vi "LWXPS_Example_GatheringCurrentNumberGet.vi"() -> ()   [LabVIEW 2013]
panel:
  out "Error out":errorcluster caption="error out"
  out "Current Number":i32
  out "Maximum Samples Number":i32
  in  "Instrument Key IN":string
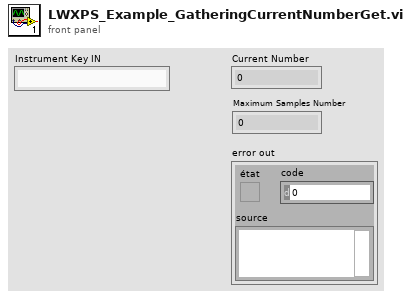
[diagram p1: front panel]
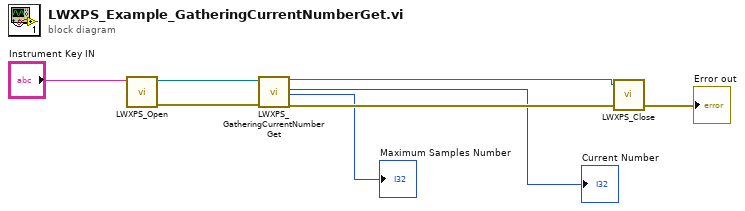
[diagram p0: block diagram]
diagram:
  n1 = call "LWXPS_Open.vi"("Instrument Key IN"="Instrument Key IN") -> ("error out"=w6:errorcluster, "CommandInterfaceXPS.XPS"=w7:refnum<k24>)  [unwired: 3 in, 2 out]
  n2 = call "LWXPS_GatheringCurrentNumberGet.vi"("XPS Reference IN"=w7, "LabVIEW error IN"=w6) -> ("CommandInterfaceXPS.XPS"=w5:refnum<k24>, "Current Number"=→"Current Number":i32, "Maximum Samples Number"=→"Maximum Samples Number":i32, "LabVIEW error OUT"=w4:errorcluster)  [unwired: 12 in, 2 out]
  n3 = call "LWXPS_Close.vi"("error in (no error)"=w4, "XPS Reference"=w5) -> ("Error out"=→"Error out":errorcluster)  [unwired: 2 in, 1 out]
